vi "Application Example.vi"() -> ()   [LabVIEW 2025, in "NewtonsPSM1735.lvlib"]
doc: "This application allow user to configure the most useful parameters of the PPA2530 and Query the Power Data"
uses:
  NewtonsPSM1735.lvlib
panel:
  in  "Integration (Signed)":u16(ring) items=["SIGNED", "MAGNITUDE"]
  out "VA Total (VA)":dbl(knob) scale=45.0..50.0
  out "Power Measurement":dbl[](array[numeric]) format="%^.4e"
  out "error out":errorcluster
  in  "Communication Interface":refnum<visa-resource-name>
  out "PF":dbl(slide) scale=0.0..1.0
  out "Frequency (Hz)":dbl(knob) scale=49.9..50.1
  out "Watt Total (W)":dbl(knob) scale=28.0..35.0
  in  "Stop Continuous Measurement":bool
  in  "Smothing response (Auto)":u16(ring) items=["AUTO", "FIXED"]
  in  "Smothing filter (Normal)":u16(ring) items=["NONE", "NORMAL", "SLOW"]
  in  "Acquisition Speed (Medium)":u16(ring) items=["FAST", "MEDIUM", "SLOW", "VERY SLOW", "WINDOW"]
  in  "Current Ranging Mode (Auto)":u16(ring) items=["AUTO", "UPAUTO", "100 mA", "316 mA", "1 A", "3,16 A", "10 A", "31,6 A", "100 A", "316 A"]
  in  "Voltage Ranging Mode (Auto)":u16(ring) items=["AUTO", "UPAUTO", "1V", "3,16V", "10V", "31,6V", "100V", "316V", "1000V", "3160V"]
  # "PSM1635\nPHASE SENSITIVE MULTIMETER"
  # "Interface Parameters"
  # "Configuration"
  # "Frequency"
  # "Hz"
  # "Watt Total"
  # "W"
  # "Watt Fondamental"
  # "W"
  # "VA"
  # "VA"
  # "VA Fundamental"
  # "W"
  # "VAR"
  # "VAR"
  # "VAR Fundamental"
  # "VAR"
  # "Power Factor"
  # "Power Factor Fundamental"
  # "Wdc"
  # "W"
  # "Harmonic Watt"
  # "W"
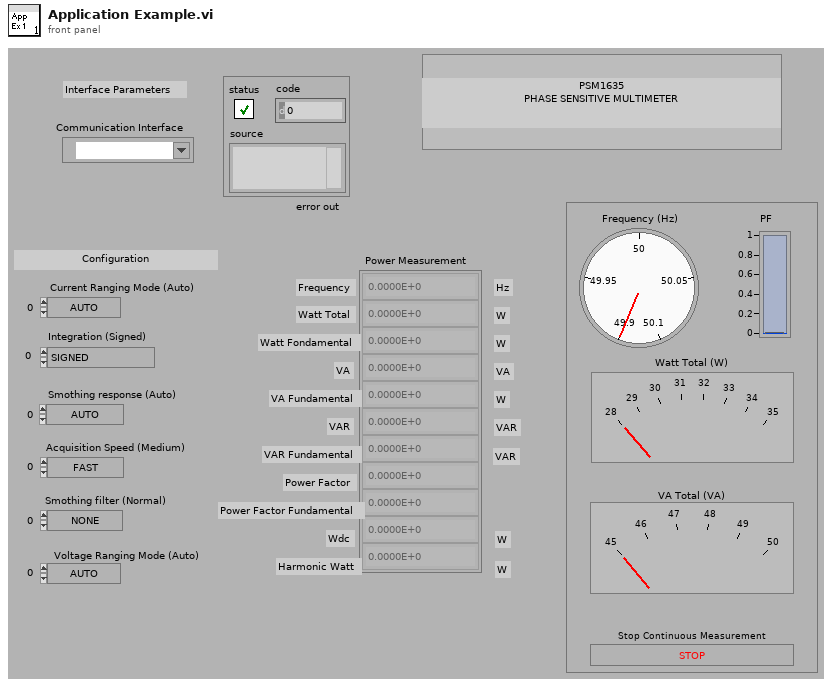
[diagram p1: front panel]
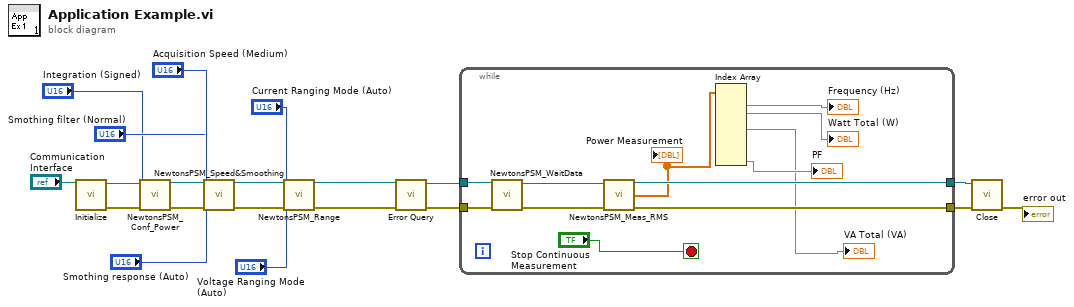
[diagram p0: block diagram]
diagram:
  n1 = call "Initialize.vi"("VISA resource name"="Communication Interface") -> ("error out"=w9:errorcluster, "VISA resource name out"=w7:refnum<visa-resource-name>)  [unwired: 4 in, 5 out]
  n2 = call "NewtonsPSM_Conf_Power.vi"("VISA session"=w7, "Integration (Signed)"="Integration (Signed)", "error in (no error)"=w9) -> ("dup VISA session"=w6:refnum<visa-resource-name>, "error out"=w8:errorcluster)  [unwired: 11 out]
  n3 = call "NewtonsPSM_Speed&Smoothing.vi"("VISA session"=w6, "Acquisition Speed (Medium)"="Acquisition Speed (Medium)", "Smothing filter (Normal)"="Smothing filter (Normal)", "Smothing response (Auto)"="Smothing response (Auto)", "error in (no error)"=w8) -> ("dup VISA session"=w15:refnum<visa-resource-name>, "error out"=w16:errorcluster)  [unwired: 5 in, 4 out]
  n4 = call "NewtonsPSM_Range.vi"("VISA session"=w15, "Input Ranging Mode (Auto)"="Voltage Ranging Mode (Auto)", "Input Input Type (Internal)"="Current Ranging Mode (Auto)", "error in (no error)"=w16) -> ("dup VISA session"=w2:refnum<visa-resource-name>, "error out"=w3:errorcluster)  [unwired: 5 in, 5 out]
  n5 = call "Error Query.vi"("error in (no error)"=w3, "VISA resource name"=w2) -> ("error out"=w4:errorcluster, "VISA resource name out"=w5:refnum<visa-resource-name>)  [unwired: 8 out]
  n6 = while {
    tunnel: [w32] -> w11
    tunnel: [w31] -> w10
    tunnel: w5 -> [w30]
    tunnel: w4 -> [w21]
    stop <- "Stop Continuous Measurement" stop-if-true
    n7 = call "NewtonsPSM_WaitData.vi"("error in (no error)"=w21, "VISA session"=w30) -> ("error out"=w28:errorcluster, "dup VISA session"=w29:refnum<visa-resource-name>)  [unwired: 6 out]
    n8 = call "NewtonsPSM_Meas_RMS.vi"("VISA session"=w29, "error in (no error)"=w28) -> ("dup VISA session"=w31:refnum<visa-resource-name>, "Measure"=w26:dbl[], "error out"=w32:errorcluster)  [unwired: 11 out]
    "Power Measurement" <- w26
    n9 = Index Array(array=w26) -> (element #1=→"Frequency (Hz)":dbl, element #2=→"Watt Total (W)":dbl, element #4=→"VA Total (VA)":dbl, element #8=→"PF":dbl)  [unwired: 8 in, 4 out]
  }
  n10 = call "Close.vi"("error in (no error)"=w11, "VISA resource name"=w10) -> ("error out"=→"error out":errorcluster)  [unwired: 9 out]
